vi "ep_Memory Init.vi"(8 "error in (no error)":errorcluster, 10 "1/previous time":dbl, 11 "1/time":dbl) -> (0 "error out":errorcluster, 2 "last memory initial value":fxp<+,51,51>, 3 "memory initial value":fxp<+,51,51>)   [LabVIEW 2012, in "NI_EP_Protection.lvlib"]
uses:
  <vilib>/addons/Electrical Power/Protection/NI_EP_Protection.lvlib
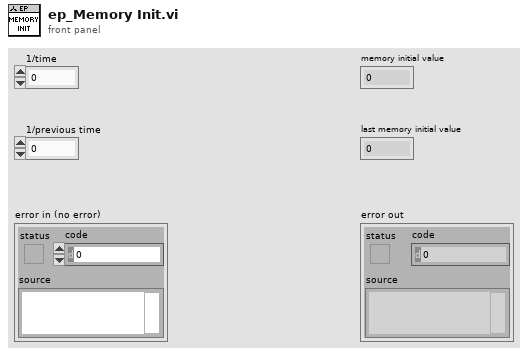
[diagram p1: front panel]
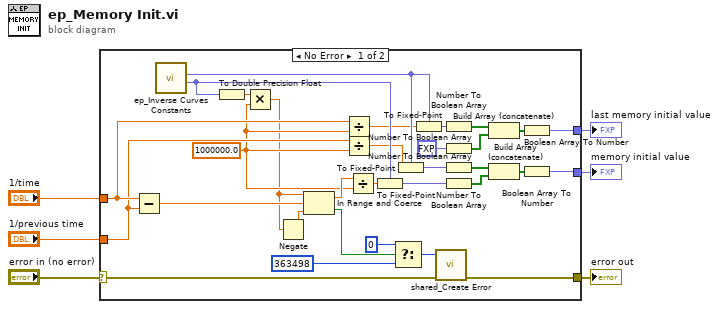
[diagram p0: block diagram]
diagram:
  n1 = case shown="No Error" "error in (no error)" {
    selector: "error in (no error)" -> [w33 w38]
    tunnel: "1/time" -> [w30 _]
    tunnel: "1/previous time" -> [w29 _]
    tunnel: [w36 w38] -> w4
    tunnel: [w32 _] -> w3
    tunnel: [w31 _] -> w1
    frame No Error {
      w9 = 1000000.0 ("y")
      n2 = Subtract(x=w30, y=w29) -> (x-y=w37:dbl)
      n3 = call <vilib>:"ep_Inverse Curves Constants.vi"() -> ("difference of 1/time"=w35:fxp<+/-,21,-17>, "1/time"=w34:fxp<+/-,30,-10>)  [unwired: 6 in, 4 out]
      n4 = To Double Precision Float(number=w35) -> (double precision float=w10:dbl)
      n5 = Multiply(x=w10, y=w9) -> (x*y=w8:dbl)
      n6 = Negate(x=w8) -> (-x=w7:dbl)
      n7 = In Range and Coerce(upper limit=w8, x=w37, lower limit=w7) -> (coerced(x)=w12:dbl, In Range?=w28:bool)
      n8 = Divide(x=w30, y=w9) -> (x/y=w14:dbl)
      n9 = Divide(x=w29, y=w9) -> (x/y=w13:dbl)
      n10 = Divide(x=w12, y=w9) -> (x/y=w11:dbl)
      n11 = To Fixed-Point(fixed-point type=w35, number=w11) -> (fixed-point=w20:fxp<+/-,21,-17>)
      n12 = Select(t=0, s=w28, f=363498 ("error code (0)")) -> (s? t:f=w25:i32)
      n13 = To Fixed-Point(fixed-point type=w34, number=w13) -> (fixed-point=w21:fxp<+/-,30,-10>)
      n14 = To Fixed-Point(fixed-point type=w34, number=w14) -> (fixed-point=w19:fxp<+/-,30,-10>)
      n15 = call <vilib>:"shared_Create Error.vi"("error in (no error)"=w33, "error code (0)"=w25) -> ("error out"=w36:errorcluster)  [unwired: 9 in]
      n16 = Number To Boolean Array(number=w19) -> (Boolean array=w17:bool[])
      n17 = Number To Boolean Array(number=fxp<+,20,2> 0.0 ("fixed-point")) -> (Boolean array=w16:bool[])
      n18 = Number To Boolean Array(number=w21) -> (Boolean array=w22:bool[])
      n19 = Number To Boolean Array(number=w20) -> (Boolean array=w23:bool[])
      n20 = Build Array (concatenate)(w17, w16) -> (w15:bool[])
      n21 = Build Array (concatenate)(w22, w23) -> (w24:bool[])
      n22 = Boolean Array To Number(Boolean array=w15) -> (number=w31:fxp<+,51,51>)
      n23 = Boolean Array To Number(Boolean array=w24) -> (number=w32:fxp<+,51,51>)
    }
    frame Error {
    }
  }
  "error out" <- w4
  "memory initial value" <- w3
  "last memory initial value" <- w1
